vi "MotorPositionController Example.vi"() -> ()   [LabVIEW 2012, in "Phidget Motor Position Controller.lvlib"]
uses:
  <instrlib>/Phidgets/Phidget Motor Position Controller/Phidget Motor Position Controller.lvlib
  <instrlib>/Phidgets/Phidget Motor Position Controller/Public/MotorPositionControllerStart.vi
  <instrlib>/Phidgets/Phidget Motor Position Controller/Public/MotorPositionControllerClose.vi
  <instrlib>/Phidgets/Phidget Common/Phidget Common.lvlib
panel:
  in  "MotorPosCtrl Init Data":T1={"Rescale Factor"=1.0, "Velocity Limit"=20000.0, "Acceleration"=10000.0, "Kp"=2000.0, "Ki"=5.0, "Kd"=25000.0, "DeadBand"=0.0}
  in  "Engaged":bool=TRUE
  out "Position":dbl
  in  "Target Position":dbl(slide) caption="Duty Cycle" scale=-100000.0..100000.0
  in  "stop":bool
  out "Duty Cycle":dbl caption="Duty Cycle Return"
  in  "Device Info":T2={"Serial Number"=-1, "Channel"=0, "Port"=0}
  out "Attached?":bool
  out "Serial Number Return":i32
  out "error out":errorcluster
  # "The default Velocity Limit and Acceleration settings seen here are not compatible with the DCC1100 BLDC Motor controller. They may both be set  to 200 (or some other compatible value) for \nthe device to work."
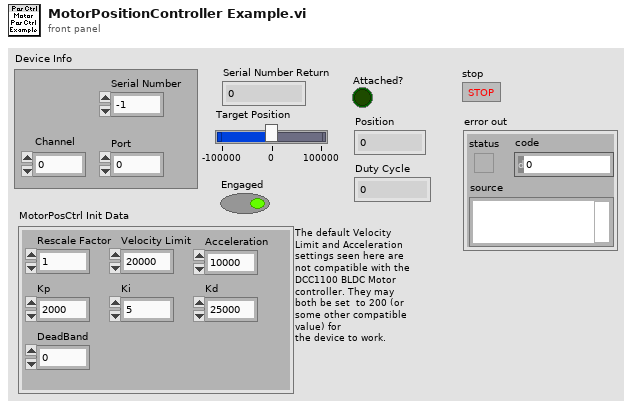
[diagram p1: front panel]
types:
  T1 = cluster{"Rescale Factor":dbl, "Velocity Limit":dbl, "Acceleration":dbl, "Kp":dbl, "Ki":dbl, "Kd":dbl, "DeadBand":dbl}
  T2 = cluster{"Serial Number":i32, "Channel":i32, "Port":i32}
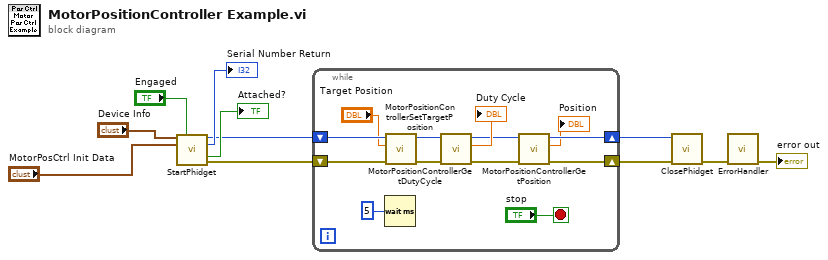
[diagram p0: block diagram]
diagram:
  n1 = call-poly <instrlib>:"StartPhidget.vi"("Device Info"="Device Info", "Engaged"="Engaged", "MotorPosCtrl Init Data"="MotorPosCtrl Init Data") -> ("Phidget ID"=w4:u64, "Serial Number Return"=→"Serial Number Return":i32, "Attached?"=→"Attached?":bool, "error out"=w3:errorcluster)  [unwired: 9 in]
  n2 = while {
    shift-right: [w15] -> w5
    shift-left: w4 -> [w19]
    shift-right: [w14] -> w6
    shift-left: w3 -> [w18]
    stop <- "stop" stop-if-true
    n3 = Wait (ms)(milliseconds to wait=u32 5) -> ()  [unwired: 1 out]
    n4 = call <instrlib>:"MotorPositionControllerSetTargetPosition.vi"("error in (no error)"=w18, "Position"="Target Position", "Device In"=w19) -> ("error out"=w21:errorcluster, "Device Out"=w20:u64)  [unwired: 6 in]
    n5 = call <instrlib>:"MotorPositionControllerGetDutyCycle.vi"("error in (no error)"=w21, "Device In"=w20) -> ("error out"=w13:errorcluster, "Duty Cycle"=→"Duty Cycle":dbl, "Device Out"=w16:u64)  [unwired: 6 in]
    n6 = call <instrlib>:"MotorPositionControllerGetPosition.vi"("error in (no error)"=w13, "Device In"=w16) -> ("error out"=w14:errorcluster, "Position"=→"Position":dbl, "Device Out"=w15:u64)  [unwired: 6 in]
  }
  n7 = call-poly <instrlib>:"ClosePhidget.vi"("error in"=w6, "Device In"=w5) -> ("error out"=w11:errorcluster)  [unwired: 9 in]
  n8 = call <instrlib>:"ErrorHandler.vi"("error in"=w11) -> ("error out"=→"error out":errorcluster)  [unwired: 9 in, 1 out]
